vi "HEWH Determine Station To Save PRAT RLT.vi"(8 "Error In":errorcluster, 10 "Array":bool[](array[boolean]), 11 "Data Loop?":bool) -> (0 "Error Out":errorcluster, 3 "SM States":string)   [LabVIEW 2019]
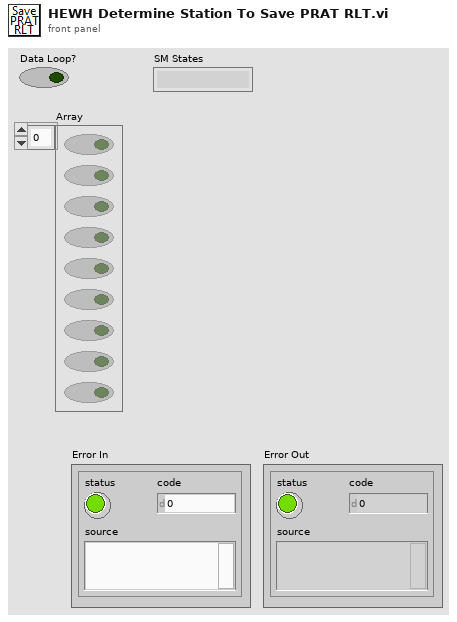
[diagram p1: front panel]
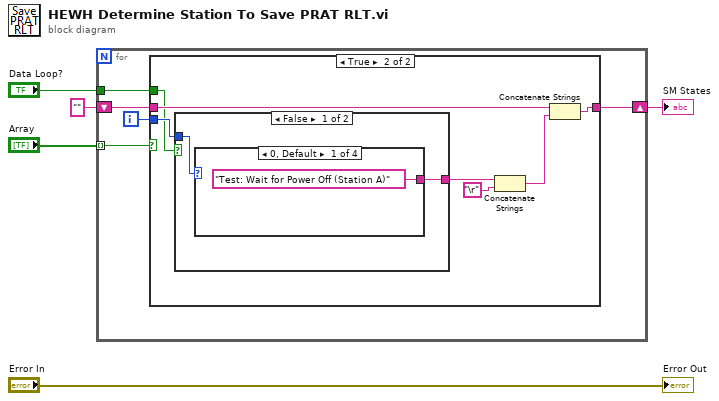
[diagram p0: block diagram]
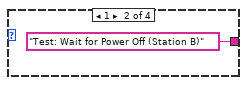
[diagram p3: hidden frame]
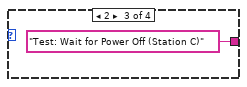
[diagram p4: hidden frame]
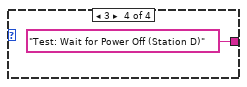
[diagram p5: hidden frame]
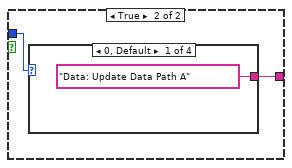
[diagram p6: hidden frame]
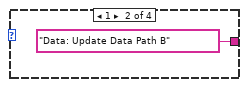
[diagram p7: hidden frame]
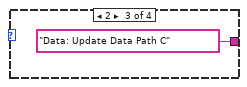
[diagram p8: hidden frame]
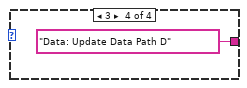
[diagram p9: hidden frame]
diagram:
  n1 = for {
    tunnel: "Array" -> [w7] mode=indexing
    shift-right: [w8] -> w4
    shift-left: "" -> [w9]
    tunnel: "Data Loop?" -> [w6]
    i -> [w10]
    n2 = case shown="True" w7 {
      tunnel: w10 -> [_ w18]
      tunnel: w9 -> [w11 w15]
      tunnel: [w11 w14] -> w8
      tunnel: w6 -> [_ w12]
      frame False {
      }
      frame True {
        n3 = case shown="False" w12 {
          tunnel: w18 -> [w19 w26]
          tunnel: [w20 w25] -> w17
          frame False {
            n4 = case shown="0, Default" w19 {
              tunnel: ["Test: Wait for Power Off (Station A)" ("State(s) at Back (\"\")") "Test: Wait for Power Off (Station B)" ("State(s) at Back (\"\")") "Test: Wait for Power Off (Station C)" ("State(s) at Back (\"\")") "Test: Wait for Power Off (Station D)" ("State(s) at Back (\"\")")] -> w20
              frame 0, Default {
              }
              frame 1 {
              }
              frame 2 {
              }
              frame 3 {
              }
            }
          }
          frame True {
            n5 = case shown="0, Default" w26 {
              tunnel: ["Data: Update Data Path A" "Data: Update Data Path B" "Data: Update Data Path C" "Data: Update Data Path D"] -> w25
              frame 0, Default {
              }
              frame 1 {
              }
              frame 2 {
              }
              frame 3 {
              }
            }
          }
        }
        n6 = Concatenate Strings(w17, "\r") -> (w16:string)
        n7 = Concatenate Strings(w15, w16) -> (w14:string)
      }
    }
  }
  "SM States" <- w4
  "Error Out" <- "Error In"
